vi "zlock_connect.vi"(6 "timeout (1s)":u32=1000, 8 "error in (no error)":errorcluster, 9 "port (7339)":i32=7339, 10 "host":string, 11 "name":string) -> (0 "error out":errorcluster, 3 "zlock":T1)   [LabVIEW 2010]
uses:
  <userlib>/BIAS2/subvis/zlock/zlock.ctl
  <vilib>/addons/zeromq/zmq_context.lvclass
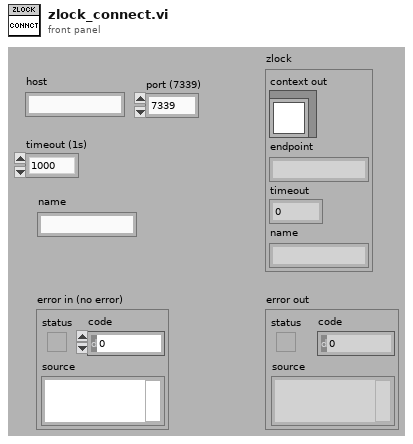
[diagram p1: front panel]
types:
  T1 = typedef "zlock.ctl" = cluster{"context out":refnum<class "zmq_context.lvclass">, "endpoint":string, "timeout":u32, "name":string}
  T2 = cluster{"context out":refnum<class "zmq_context.lvclass">, string, "timeout (1s)":u32, "name":string}
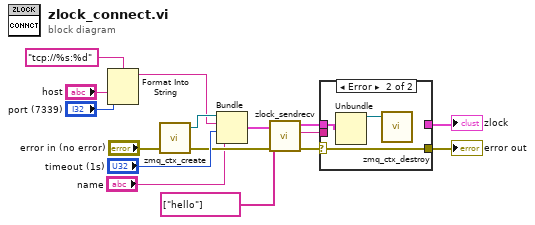
[diagram p0: block diagram]
diagram:
  n1 = Format Into String(format string="tcp://%s:%d", "host", "port (7339)") -> (resulting string=w10:string)  [unwired: 2 in, 1 out]
  n2 = call <vilib>:"zmq_ctx_create.vi"("error in"="error in (no error)") -> ("error out"=w8:errorcluster, "context out"=w16:refnum<class "zmq_context.lvclass">)  [unwired: 3 in]
  n3 = Bundle("context out"=w16, w10, "timeout (1s)"="timeout (1s)", "name"="name") -> (w5:T2)  [unwired: 1 in]
  n4 = call <userlib>:"zlock_sendrecv.vi"("error in (no error)"=w8, "parts"=string[] ["hello"], "socket in"=w5) -> ("error out"=w7:errorcluster, "reply"=w6:string, "socket out"=w4:T1)  [unwired: 6 in]
  n5 = case shown="Error" w7 {
    selector: w7 -> [w17 w19]
    tunnel: w6 -> [_ _]
    tunnel: w4 -> [w18 w21]
    tunnel: [w18 _] -> w3
    tunnel: [w17 w19] -> w2
    frame No Error {
    }
    frame Error {
      n6 = Unbundle(w21) -> ("context out"=w20:refnum<class "zmq_context.lvclass">)  [unwired: 3 out]
      n7 = call <vilib>:"zmq_ctx_destroy.vi"("context in"=w20) -> ()  [unwired: 4 in, 1 out]
    }
  }
  "error out" <- w2
  "zlock" <- w3
